vi "Read Recurrence Type.vi"(8 "error in (no error)":errorcluster, 11 "Daily in":refnum<class "Daily.lvclass">) -> (0 "error out":errorcluster, 2 "Recurrence Type":T1, 3 "Daily out":refnum<class "Daily.lvclass">)   [LabVIEW 2020, in "Daily.lvclass"]
uses:
  Daily.lvclass
  Daily.lvclass/Daily.ctl
  Daily Recurrence Type TYP.ctl
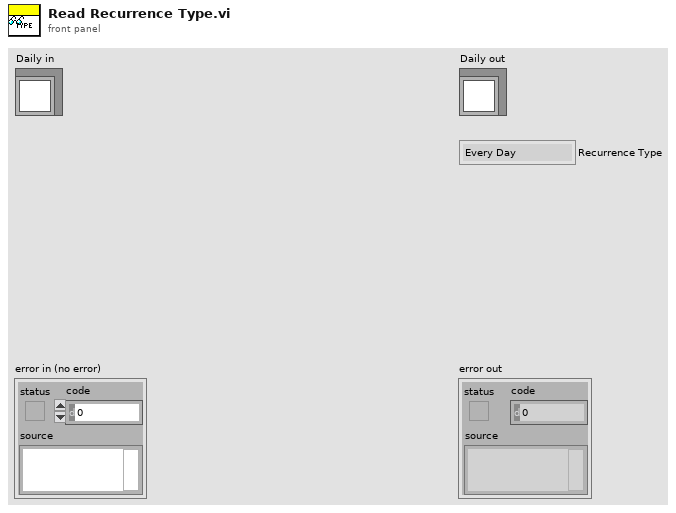
[diagram p1: front panel]
types:
  T1 = typedef "Daily.lvclass/Daily Recurrence Type TYP.ctl" = enum16{"Every Day", "Only Certain Days of the Week"}
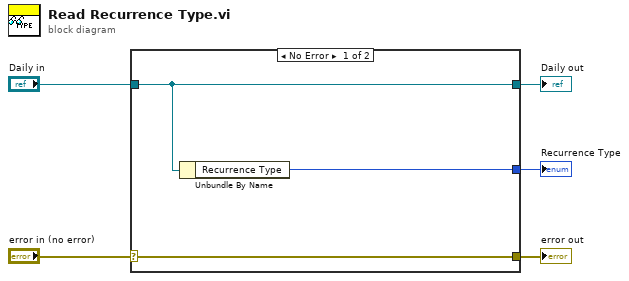
[diagram p0: block diagram]
diagram:
  n1 = case shown="No Error" "error in (no error)" {
    selector: "error in (no error)" -> [w8 w9]
    tunnel: [w8 w9] -> w4
    tunnel: [w7 w10] -> w2
    tunnel: "Daily in" -> [w7 w10]
    tunnel: [w6 _] -> w1
    frame No Error {
      n2 = Unbundle By Name(w7) -> ("Recurrence Type"=w6:T1)
    }
    frame Error {
    }
  }
  "error out" <- w4
  "Daily out" <- w2
  "Recurrence Type" <- w1
